vi "member login.vi"() -> (0 "Numeric":i32, 1 "Pass?":bool, 2 "Username":string, 3 "Password":string)   [LabVIEW 2014]
uses:
  <vilib>/Utility/file.llb/Read From Spreadsheet File (string).vi
panel:
  out "Read file path":path
  in  "OK Button":bool
  in  "Password":string
  in  "Username":string
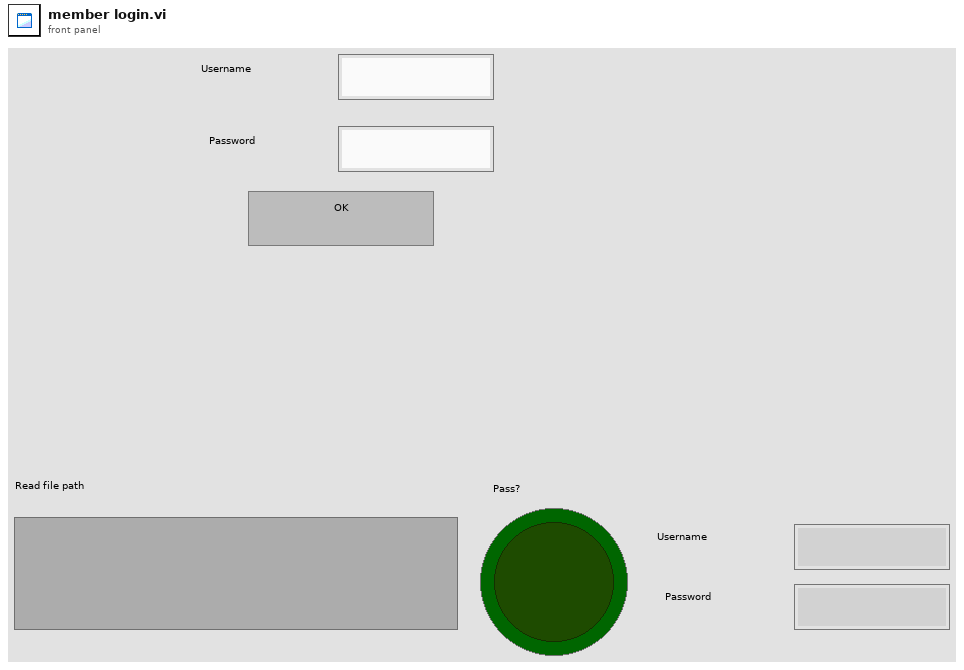
[diagram p1: front panel]
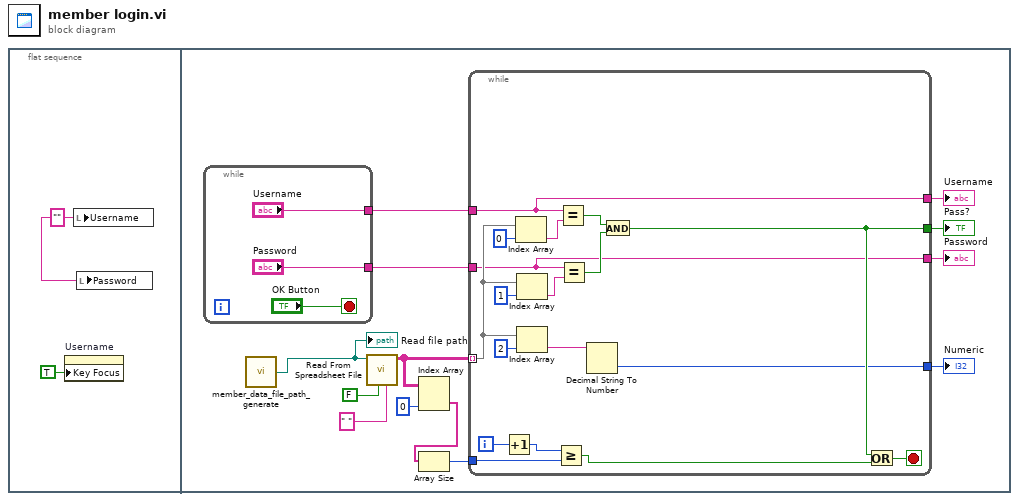
[diagram p0: block diagram]
diagram:
  n1 = flat-sequence {
    frame #0 {
      w1 = "" ("Username")
      n2 = property on="Username" class="Str"("Key Focus"=TRUE) -> ()  [unwired: 2 in, 2 out]
      n3 = local write "Username"(w1) -> ()
      n4 = local write "Password"(w1) -> ()
    }
    frame #1 {
      n5 = while {
        tunnel: ["Username"] -> w9
        tunnel: ["Password"] -> w8
        stop <- "OK Button" stop-if-true
      }
      n6 = call "member_data_file_path_generate.vi"() -> ("appended path"=w3:path)
      "Read file path" <- w3
      n7 = call-poly <vilib>:"Read From Spreadsheet File.vi"("delimiter (\\t)"=" ", "transpose (no:F)"=FALSE, "file path (dialog if empty)"=w3) -> ("all rows"=w13:string[][])  [unwired: 4 in, 4 out]
      n8 = Index Array(array=w13, index (col)=0 ("disabled index (col)")) -> (element=w11:string[])  [unwired: 1 in]
      n9 = Array Size(array=w11) -> (size(s)=w10:i32)
      n10 = while {
        tunnel: w13 -> [w20] mode=indexing
        tunnel: w10 -> [w31]
        tunnel: w9 -> [w17]
        tunnel: w8 -> [w16]
        tunnel: [w22] -> w7
        tunnel: [w18] -> w6
        tunnel: [w17] -> w5
        tunnel: [w16] -> w4
        i -> [w33]
        stop <- w24 stop-if-true
        n11 = Increment(x=w33) -> (x+1=w32:i32)
        n12 = Index Array(array=w20, index=0) -> (element=w30:string)
        n13 = Index Array(array=w20, index=1) -> (element=w28:string)
        n14 = Index Array(array=w20, index=2) -> (element=w19:string)
        n15 = Greater Or Equal?(x=w32, y=w31) -> (x >= y?=w23:bool)
        n16 = Equal?(x=w17, y=w30) -> (x = y?=w26:bool)
        n17 = Equal?(x=w16, y=w28) -> (x = y?=w25:bool)
        n18 = Decimal String To Number(string=w19) -> (number=w18:i32)  [unwired: 2 in, 1 out]
        n19 = And(x=w26, y=w25) -> (x .and. y?=w22:bool)
        n20 = Or(x=w22, y=w23) -> (x .or. y?=w24:bool)
      }
      "Pass?" <- w7
      "Numeric" <- w6
      "Username" <- w5
      "Password" <- w4
    }
  }
